vi "Autocross(2Lap).vi"() -> ()   [LabVIEW 2017]
uses:
  Control/AutocrossBestRecordIndicator.ctl
  Control/AutocrossCurrentRecordIndicator(2Lap).ctl
  Control/AutocrossState.ctl
  <vilib>/DAQmx/read.llb/DAQmx Read (Analog DBL 1Chan 1Samp).vi
  <vilib>/DAQmx/write.llb/DAQmx Write (Analog DBL 1Chan 1Samp).vi
  <vilib>/Utility/file.llb/Read Delimited Spreadsheet (string).vi
  <vilib>/DAQmx/create/channels.llb/DAQmx Create Channel (AO-Voltage-Basic).vi
  <vilib>/DAQmx/create/channels.llb/DAQmx Create Channel (AI-Voltage-Basic).vi
panel:
  out "Event Progress":string[][](table)
  in  "DeviceName":tag
  in  "OK Button":bool
  in  "Ready":bool
  in  "Retry":bool
  out "CurrentRecordIndicator":T1
  out "BestRecordIndicator":T2
  in  "Stop":bool
  # "2019 KSAE Formula Autocross Event"
  # "Lap1:"
  # "Lap2:"
  # "Total:"
  # "Entry:"
  # "#1"
  # "#2"
  # "#3"
  # "#4"
  # "Univ. :"
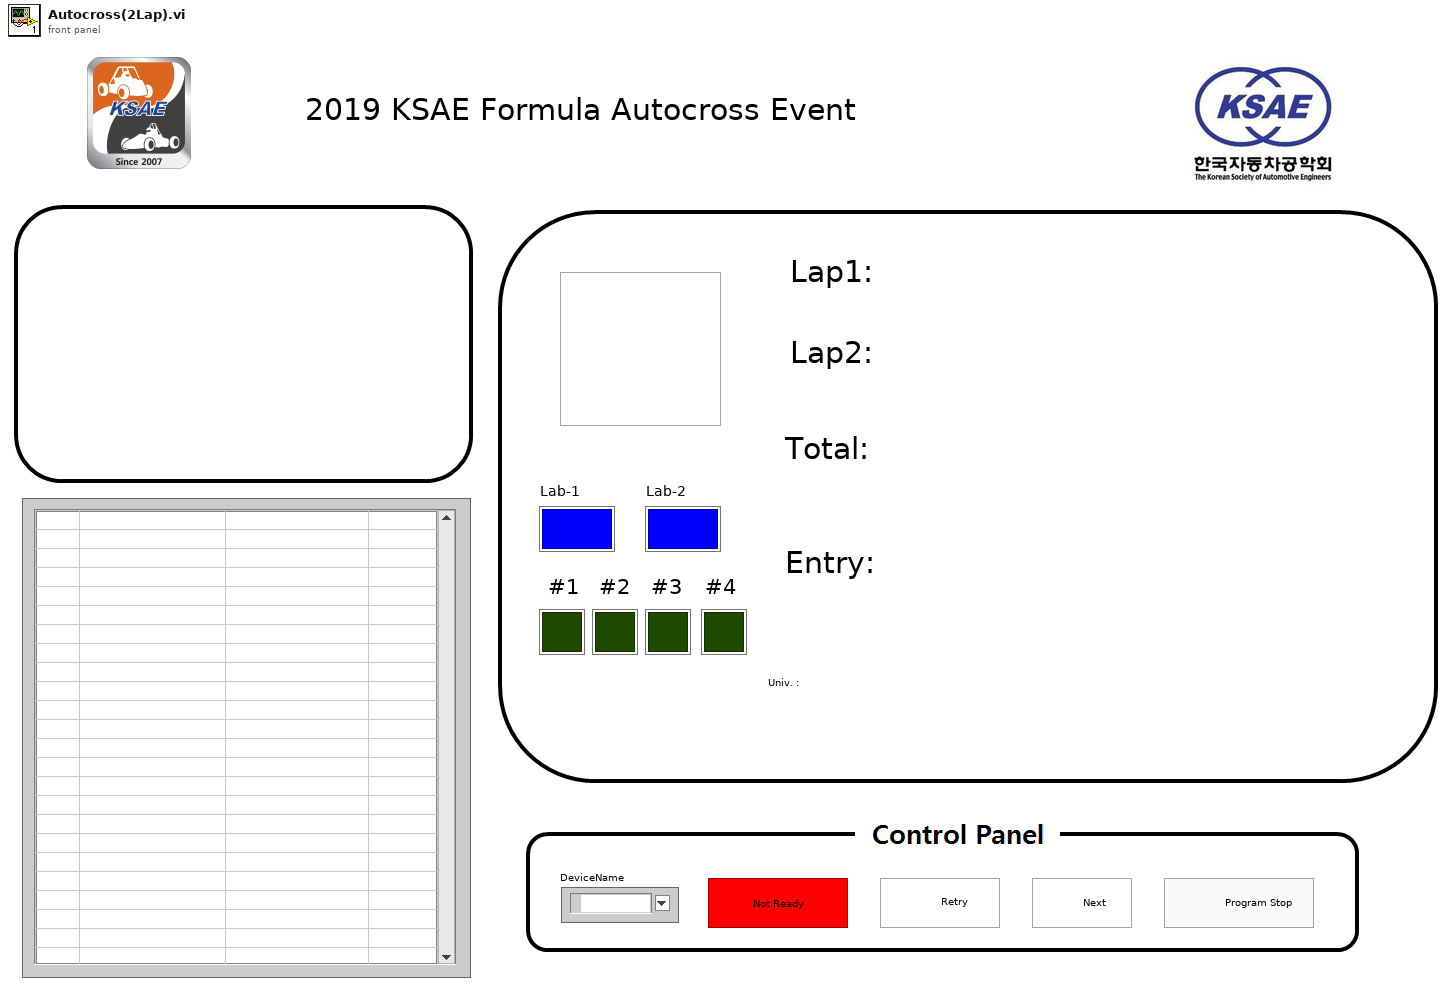
[diagram p1: front panel]
types:
  T1 = typedef "AutocrossCurrentRecordIndicator(2Lap).ctl" = cluster{"Lab1":string, "Lab2":string, "TotalLabTime":string, "CurrentEntry":string, "CurrentUniversity":string, "Flag":picture, "CurrentState":string, "LapProgress":cluster{"Lab-1":bool, "Lab-2":bool}, "EventCount":cluster{"Attempt-1":bool, "Attempt-2":bool, "Attempt-3":bool, "Attempt-4":bool}}
  T2 = typedef "AutocrossBestRecordIndicator.ctl" = cluster{"BestSchool":string, "BestEntry":string, "BestTime":string}
  T3 = typedef "AutocrossState.ctl" = enum16{"Initial", "InputInfomation", "Ready", "1lap", "2lap", "FinshRunning", "LogRecord", "RenewBestRecord", "ProgramStop"}
  T4 = cluster{"CurrentRecordIndicator":T1, "BestRecordIndicator":T2, "FlageData":cluster{"GreenFlag":picture, "BlueFlag":picture, "RedFlag":picture}, "1LapTime":i64, "2LapTime":i64, "TotalLabTime":i64, "InternalTime(1Lap)":i64, "InternalTime(2Lap)":i64, "State":T3, "EventProgressData":string[][], "EventCount":i32}
  T5 = cluster{"Attempt-1":bool, "Attempt-2":bool, "Attempt-3":bool, "Attempt-4":bool}
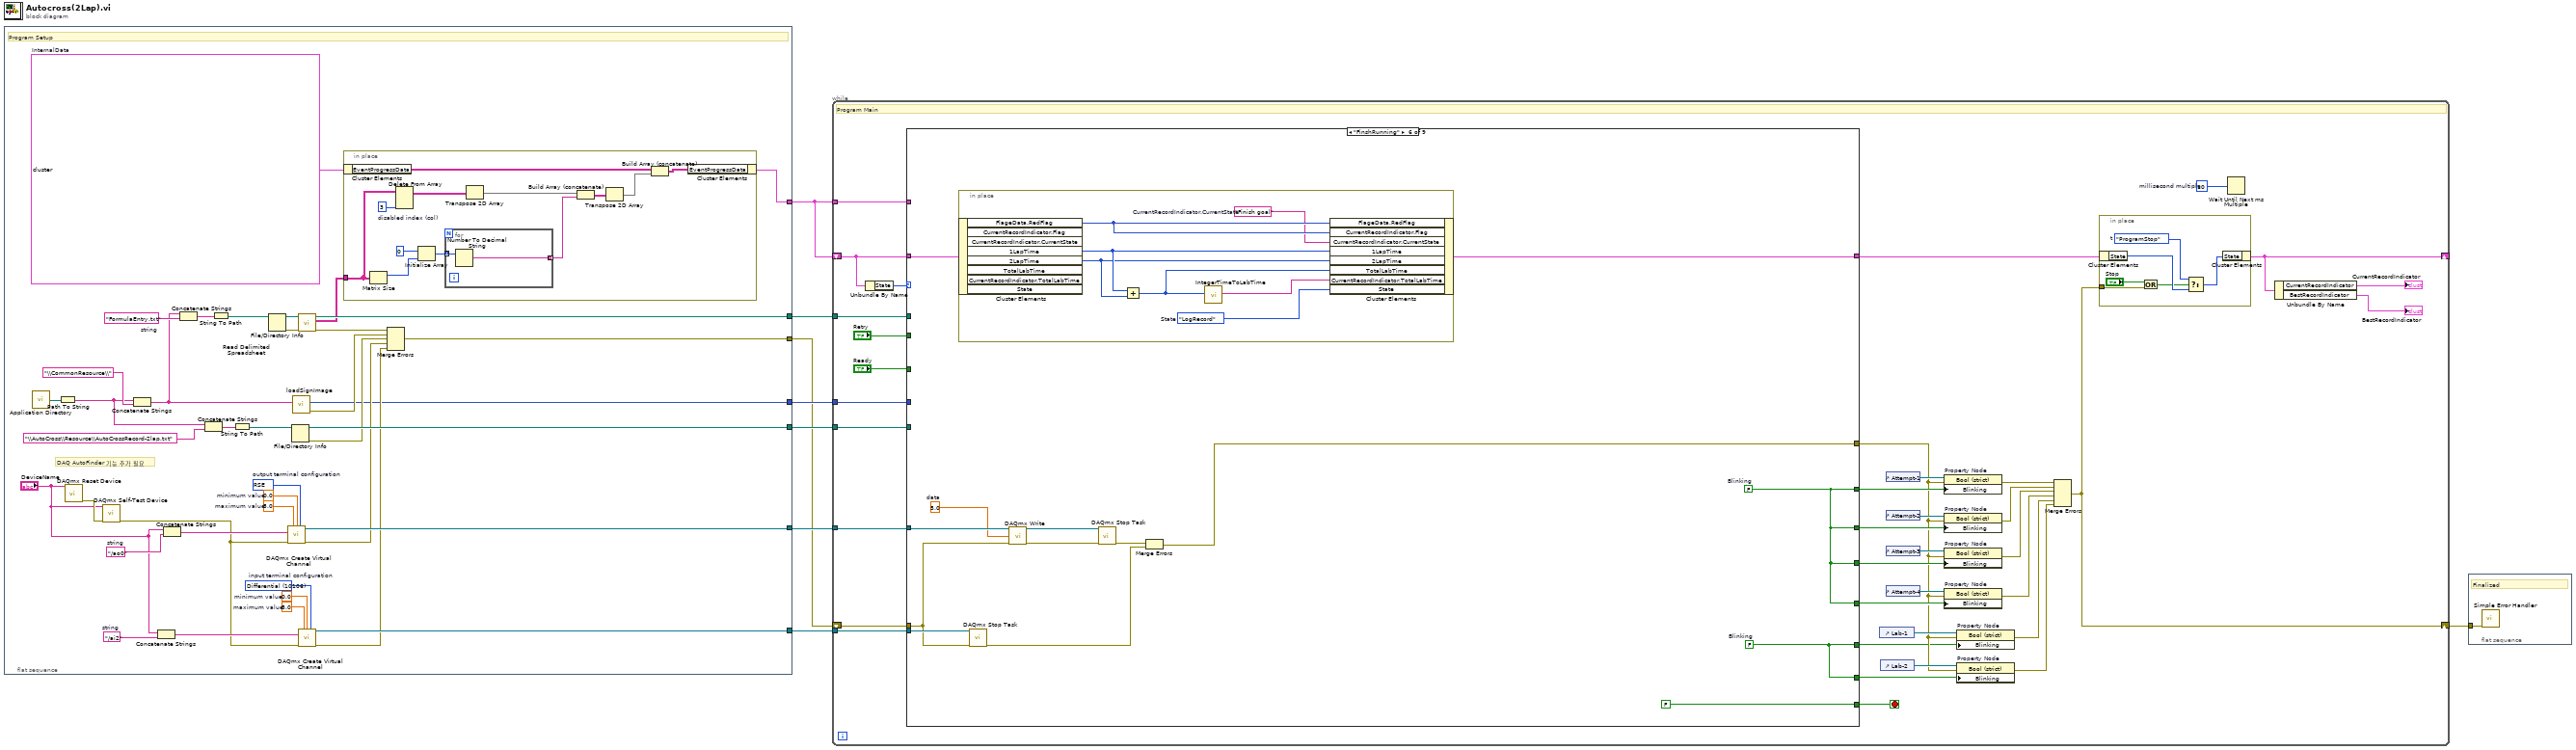
[diagram p0: block diagram]
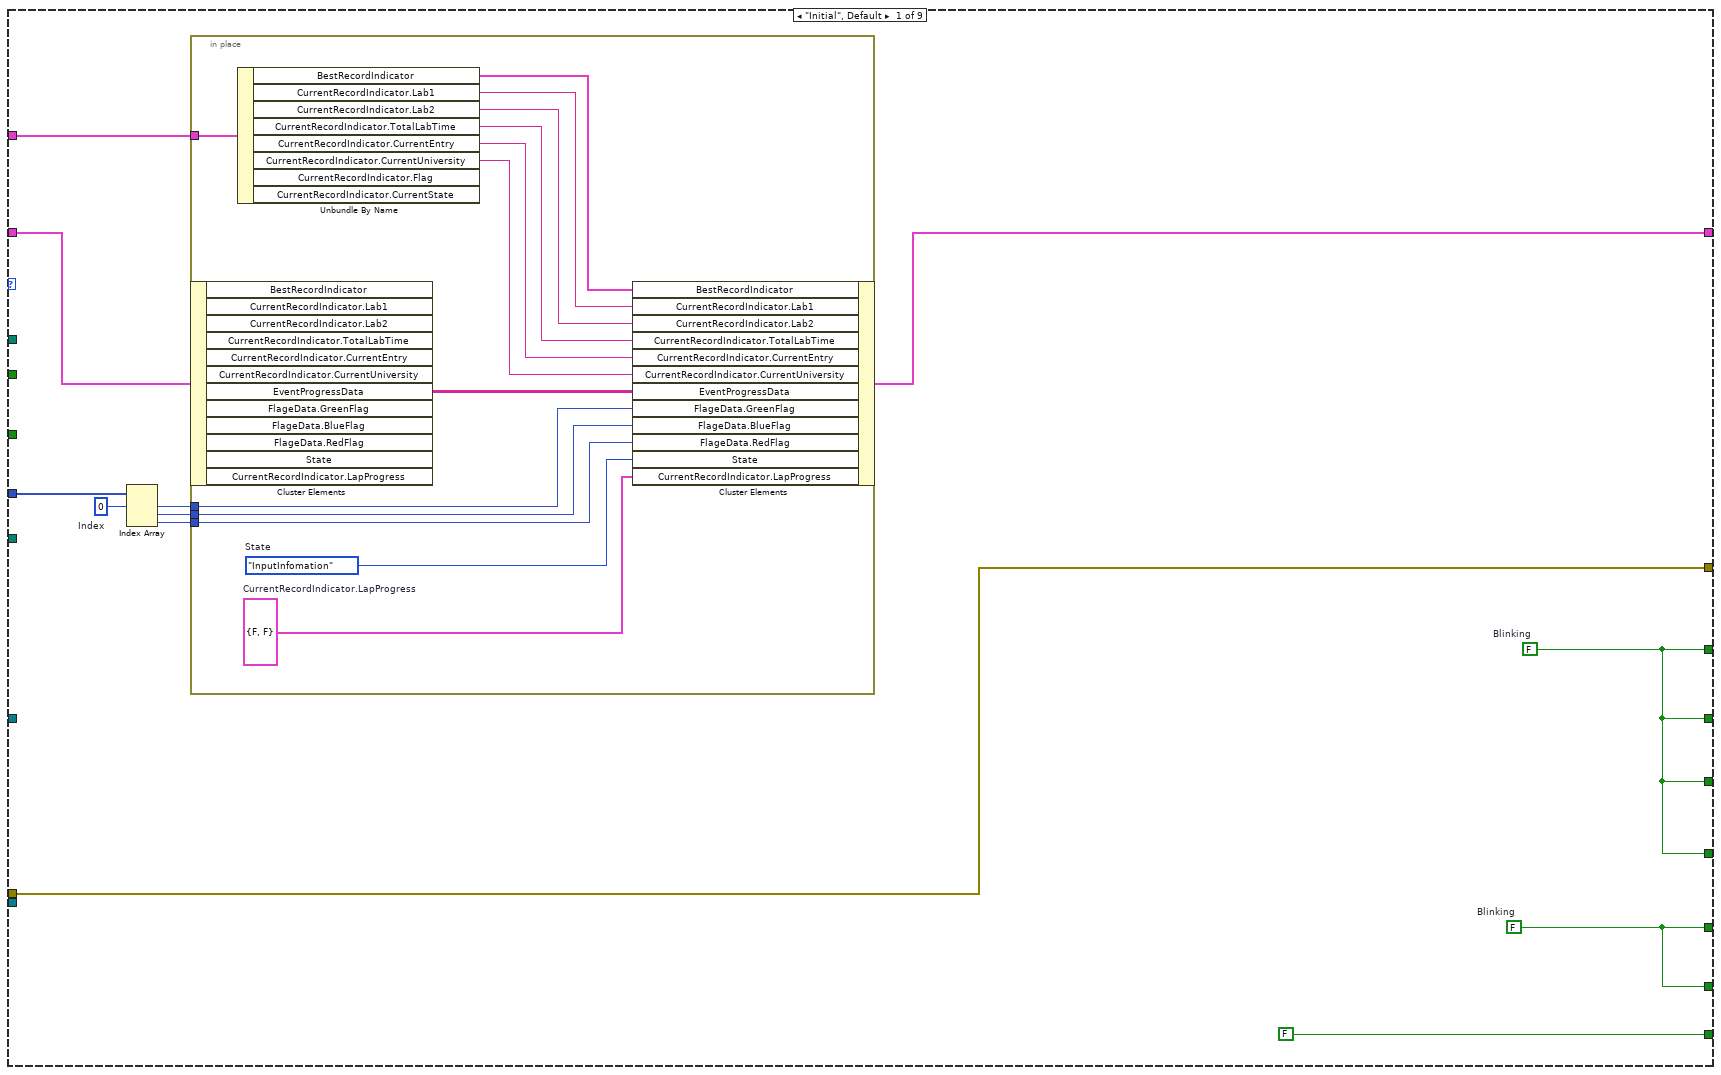
[diagram p2: hidden frame]
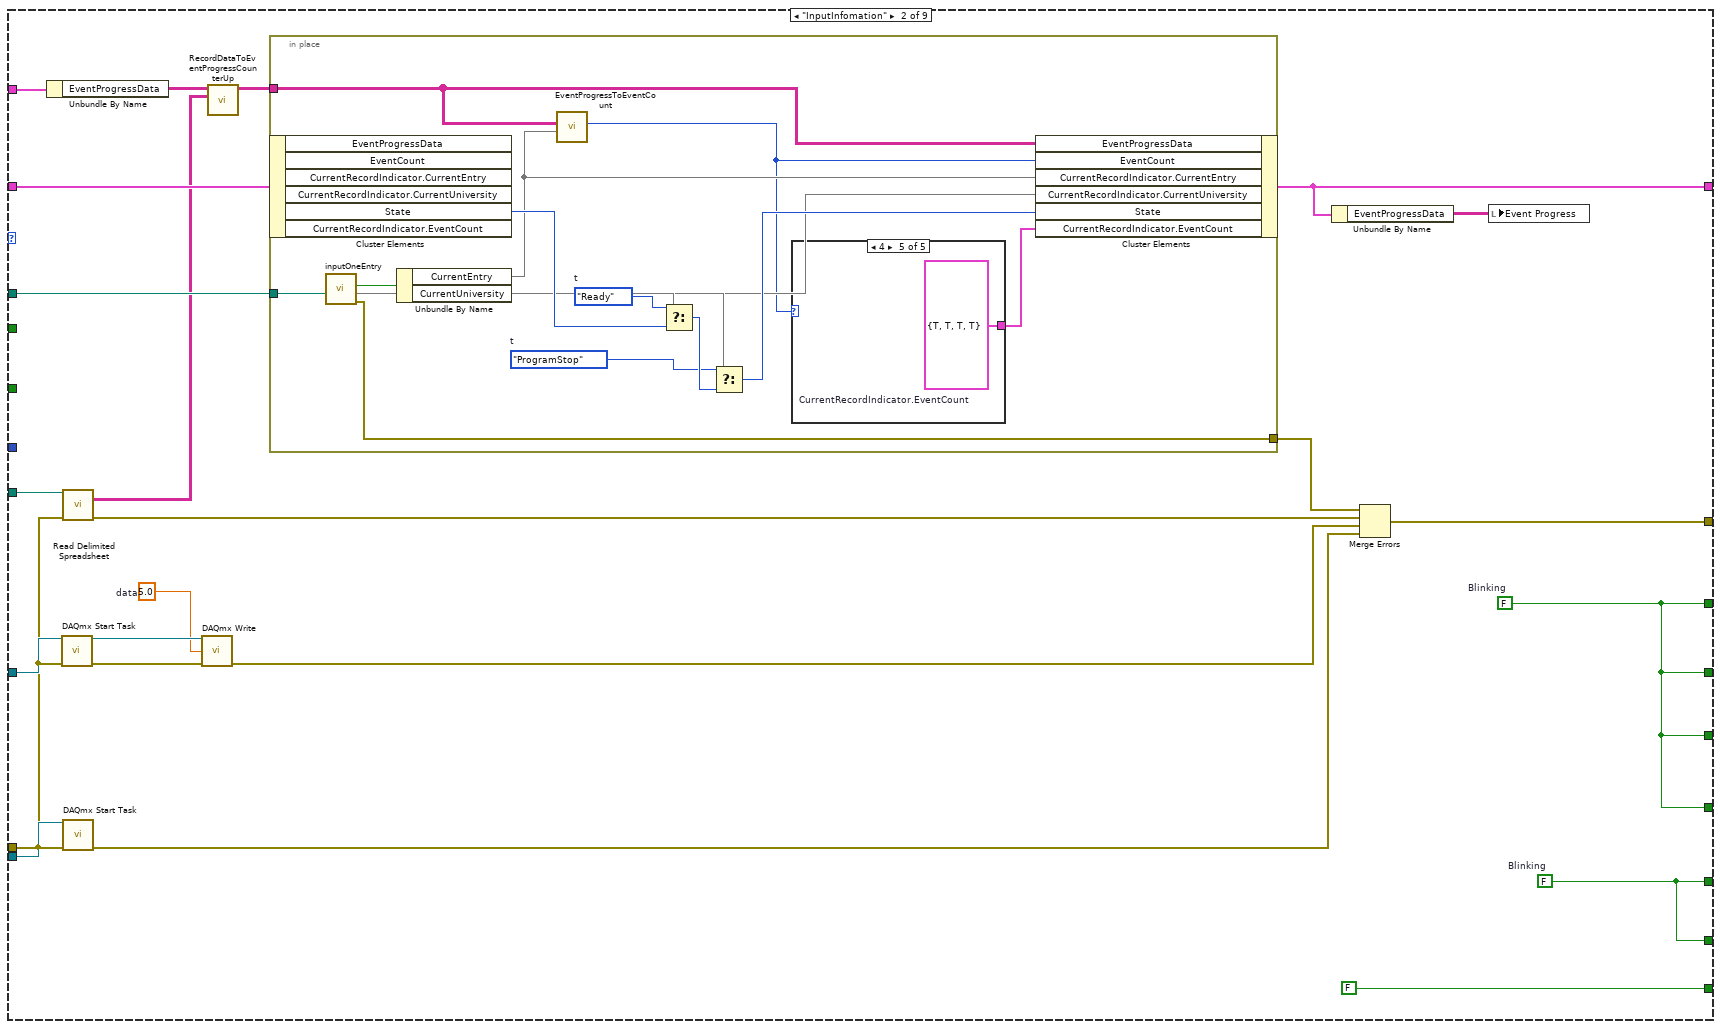
[diagram p3: hidden frame]
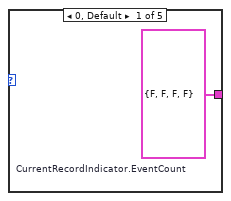
[diagram p4: hidden frame]
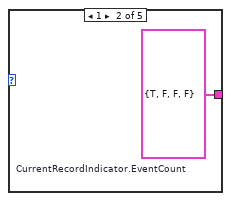
[diagram p5: hidden frame]
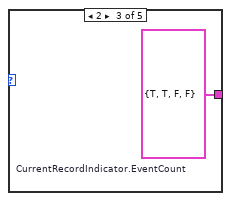
[diagram p6: hidden frame]
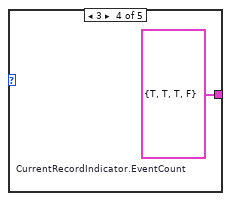
[diagram p7: hidden frame]
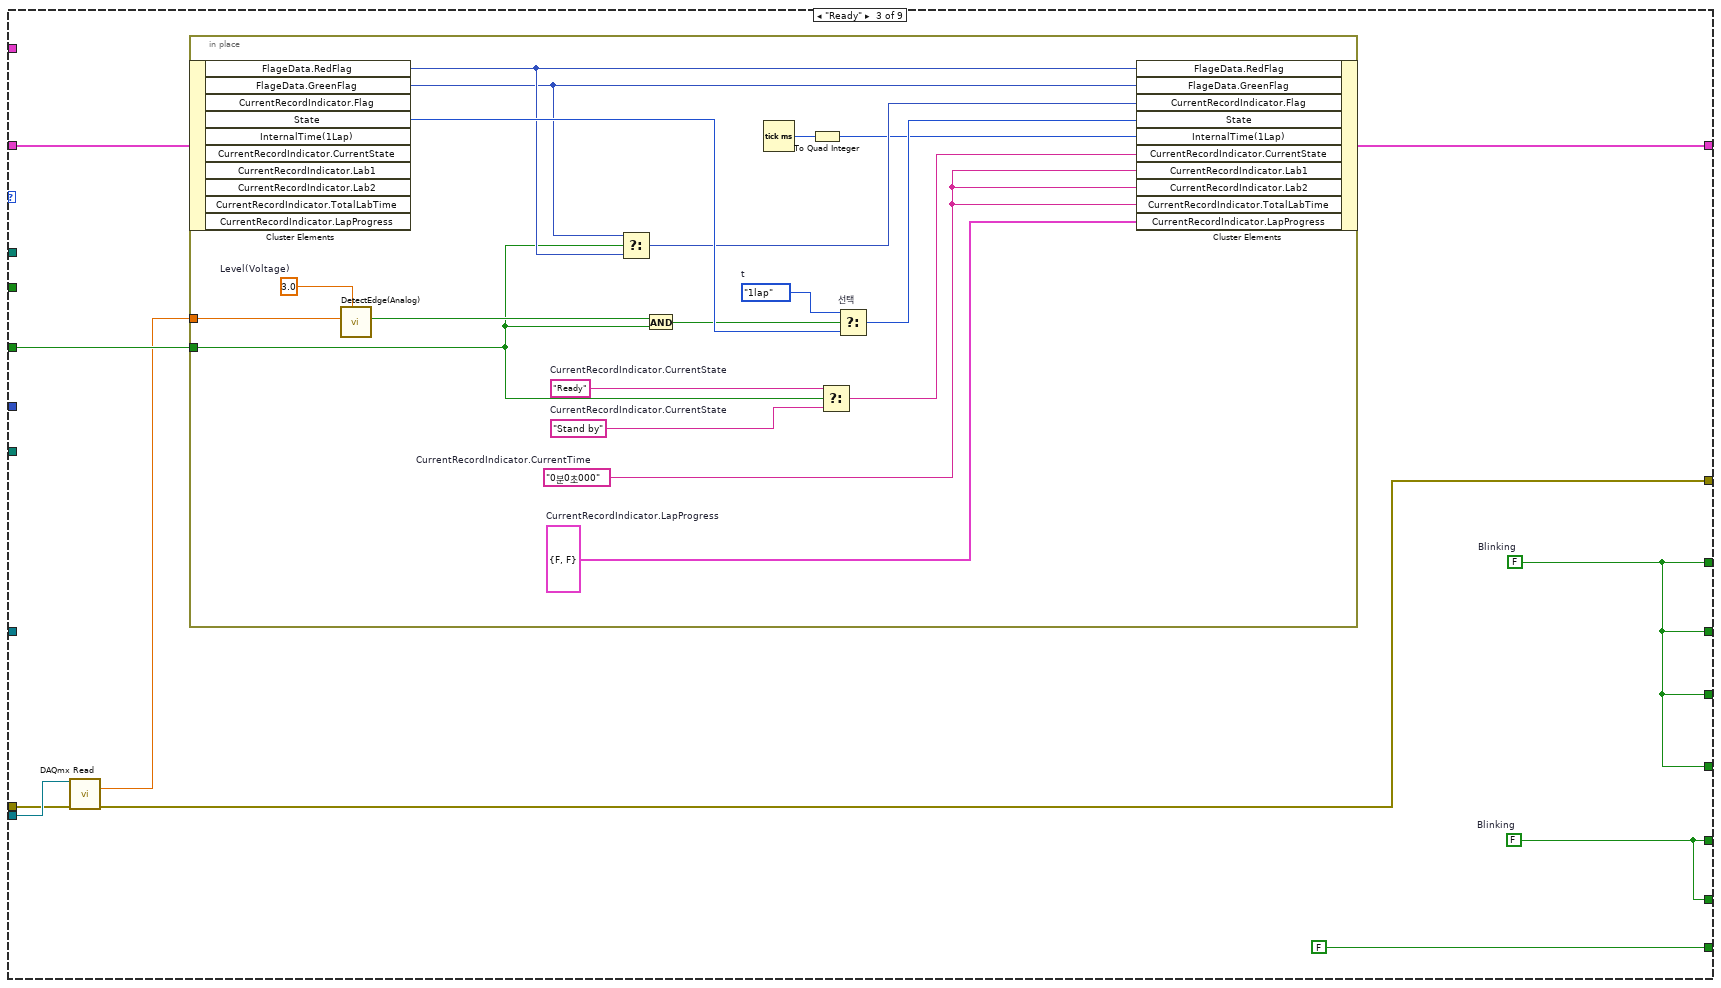
[diagram p8: hidden frame]
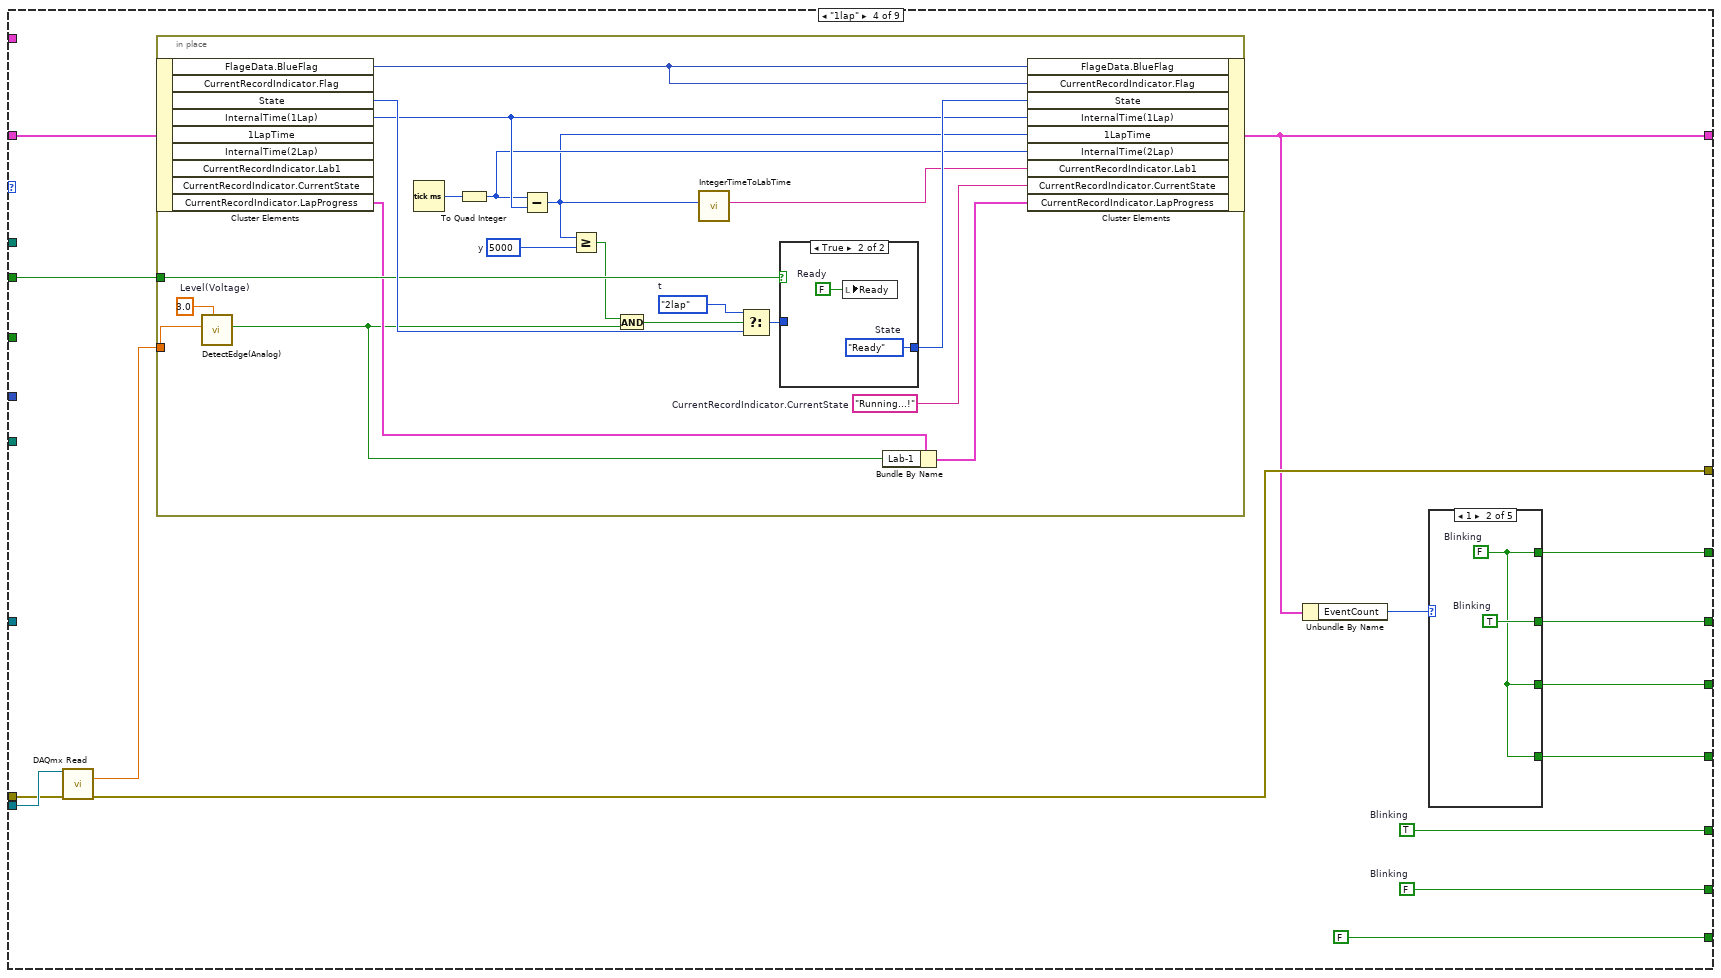
[diagram p9: hidden frame]
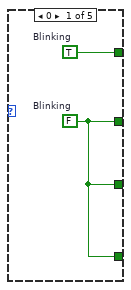
[diagram p10: hidden frame]
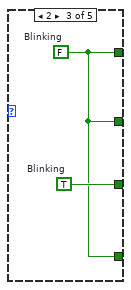
[diagram p11: hidden frame]
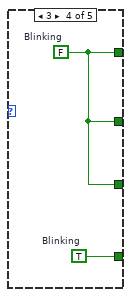
[diagram p12: hidden frame]
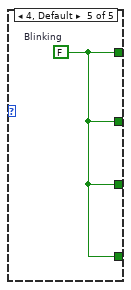
[diagram p13: hidden frame]
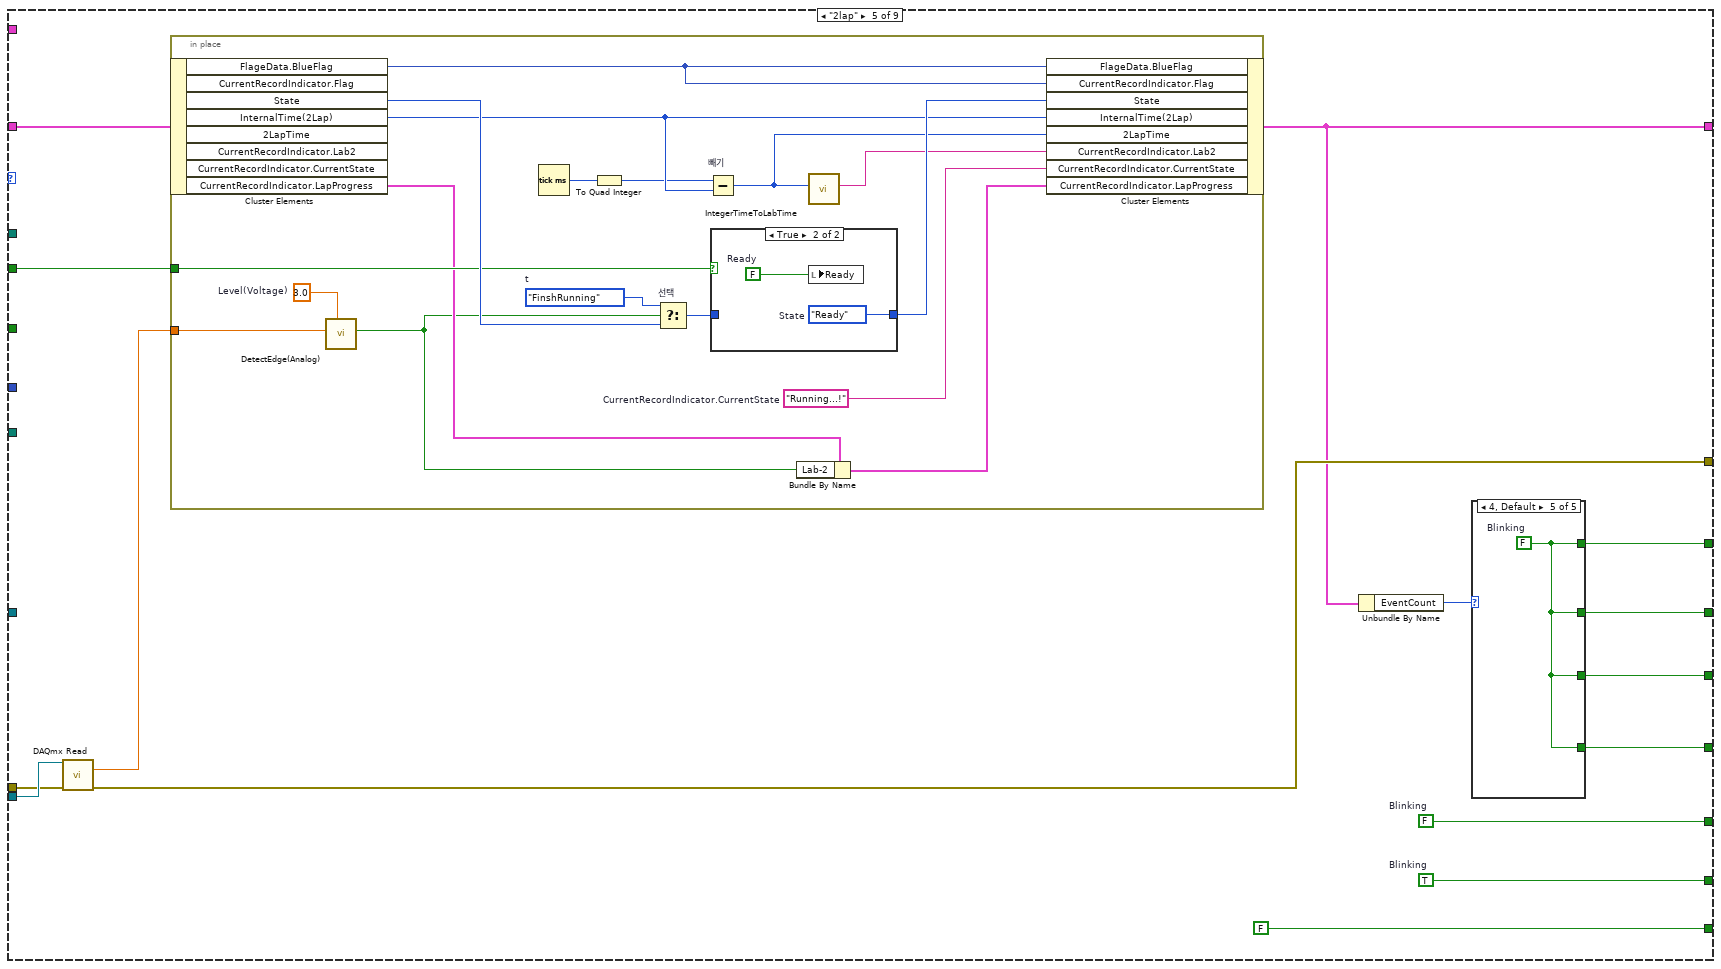
[diagram p15: hidden frame]
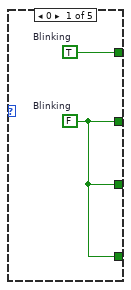
[diagram p16: hidden frame]
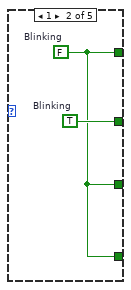
[diagram p17: hidden frame]
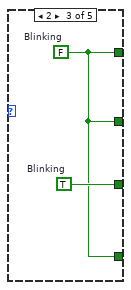
[diagram p18: hidden frame]
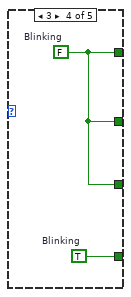
[diagram p19: hidden frame]
diagram:
  n1 = flat-sequence {
    tunnel: [w23] -> w7
    tunnel: [w46] -> w6
    tunnel: [w43] -> w5
    tunnel: [w25] -> w4
    tunnel: [w16] -> w3
    tunnel: [w9] -> w2
    tunnel: [w18] -> w1
    frame #0 {
      w24 = T4 {"CurrentRecordIndicator"={"Lab1"="", "Lab2"="", "TotalLabTime"="", "CurrentEntry"="", "CurrentUniversity"="", "Flag"=bytes[0], "CurrentState"="", "LapProgress"={"Lab-1"=FALSE, "Lab-2"=FALSE}, "EventCount"={"Attempt-1"=FALSE, "Attempt-2"=FALSE, "Attempt-3"=FALSE, "Attempt-4"=FALSE}}, "BestRecordIndicator"={"BestSchool"="", "BestEntry"="", "BestTime"=""}, "FlageData"={"GreenFlag"=bytes[0], "BlueFlag"=bytes[0], "RedFlag"=bytes[0]}, "1LapTime"=0, "2LapTime"=0, "TotalLabTime"=0, "InternalTime(1Lap)"=0, "InternalTime(2Lap)"=0, "State"=enum."Initial", "EventProgressData"=[["Entry ", "University", "Team", "Event Run "]], "EventCount"=0}  # InternalData
      w31 = "/ai2"  # string
      w32 = "/ao0"  # string
      w33 = "FormulaEntry.txt"  # string
      w40 = 10083 items=["Default"=-1, "RSE"=10083, "Differential"=10106, "Pseudodifferential"=12529]  # output terminal configuration
      w41 = 0.0  # minimum value
      w42 = 5.0  # maximum value
      w45 = 5.0  # maximum value
      w44 = 0.0  # minimum value
      w47 = 10106 items=["default"=-1, "RSE"=10083, "NRSE"=10078, "Differential"=10106, "Pseudodifferential"=12529]  # input terminal configuration
      # "DAQ AutoFinder 기능 추가 필요"
      # "Program Setup"
      n2 = call <vilib>:"Application Directory.vi"() -> ("Application Directory"=w39:path)
      n3 = Path To String(path=w39) -> (string=w35:string)
      n4 = call <vilib>:"DAQmx Reset Device.vi"("device in"="DeviceName") -> ("error out"=w12:errorcluster)  [unwired: 14 in]
      n5 = call <vilib>:"DAQmx Self-Test Device.vi"("device in"="DeviceName", "error in"=w12) -> ("error out"=w10:errorcluster)  [unwired: 13 in]
      n6 = Concatenate Strings "Concatenate Strings"(w35, "\\CommonResource\\") -> (w27:string)
      n7 = Concatenate Strings "Concatenate Strings"("DeviceName", w31) -> (w29:string)
      n8 = Concatenate Strings "Concatenate Strings"("DeviceName", w32) -> (w30:string)
      n9 = Concatenate Strings "Concatenate Strings"(w27, w33) -> (w34:string)
      n10 = Concatenate Strings "Concatenate Strings"(w35, "\\AutoCross\\Resource\\AutoCrossRecord-2lap.txt") -> (w37:string)
      n11 = String To Path(string=w34) -> (path=w26:path)
      n12 = String To Path(string=w37) -> (path=w28:path)
      n13 = File/Directory Info(path=w26) -> (path out=w17:path, error out=w15:errorcluster)  [unwired: 1 in, 5 out]
      n14 = call-poly <vilib>:"DAQmx Create Virtual Channel.vi"("maximum value"=w42, "minimum value"=w41, "output terminal configuration"=w40, "physical channels"=w30, "error in"=w10) -> ("task out"=w43:refnum<k21>, "error out"=w20:errorcluster)  [unwired: 9 in]
      n15 = File/Directory Info(path=w28) -> (path out=w25:path, error out=w21:errorcluster)  [unwired: 1 in, 5 out]
      n16 = call "loadSignImage.vi"("String"=w27) -> ("outputError"=w22:errorcluster, "SignImageOutput"=w9:picture[])  [unwired: 9 in]
      n17 = call-poly <vilib>:"Read Delimited Spreadsheet.vi"("file path (dialog if empty)"=w17, "error in (no error)"=w15) -> ("new file path (Not A Path if cancelled)"=w16:path, "all rows"=w13:string[][], "error out"=w14:errorcluster)  [unwired: 8 in, 3 out]
      n18 = call-poly <vilib>:"DAQmx Create Virtual Channel.vi"("maximum value"=w45, "minimum value"=w44, "input terminal configuration"=w47, "physical channels"=w29, "error in"=w10) -> ("task out"=w46:refnum<k21>, "error out"=w19:errorcluster)  [unwired: 9 in]
      n19 = in-place {
        in-place-border: w13 -> [w48]
        w56 = 3  # disabled index (col)
        n20 = in-place-cluster #1(w24) -> ("EventProgressData"=w50:string[][])
        n21 = Matrix Size(0:w48) -> (1:w59:i32)  [unwired: 1 out]
        n22 = Delete From Array "Delete From Array"(array=w48, index (col)=w56) -> (array with subset deleted=w55:string[][])  [unwired: 2 in, 1 out]
        n23 = Initialize Array "Initialize Array"(0, w59) -> (w57:i32[])
        n24 = for {
          tunnel: w57 -> [w61] mode=indexing
          tunnel: [w60] -> w53 mode=indexing
          n25 = Number To Decimal String(number=w61) -> (decimal integer string=w60:string)  [unwired: 1 in]
        }
        n26 = Transpose 2D Array(2D array=w55) -> (transposed array=w54:string[][])
        n27 = Build Array (concatenate) "Build Array"(w54, w53) -> (w52:string[][])
        n28 = Transpose 2D Array(2D array=w52) -> (transposed array=w51:string[][])
        n29 = Build Array (concatenate) "Build Array"(w50, w51) -> (w49:string[][])
        n30 = in-place-cluster #1("EventProgressData"=w49) -> (w23:T4)
      }
      n31 = Merge Errors "Merge Errors"(w14, w22, w21, w20, w19) -> (w18:errorcluster)
    }
  }
  n32 = while {
    tunnel: w6 -> [w98]
    shift-right: [w91] -> _
    shift-left: w7 -> [w95]
    shift-right: [w69] -> w8
    shift-left: w1 -> [w97]
    tunnel: w7 -> [w89]
    tunnel: w5 -> [w86]
    tunnel: w4 -> [w85]
    tunnel: w3 -> [w84]
    tunnel: w2 -> [w82]
    stop <- w90 stop-if-true
    w83 = u32 10  # millisecond multiple
    # "Program Main"
    n33 = Unbundle By Name(w95) -> ("State"=w96:T3)
    n34 = case shown="\"FinshRunning\"" w96 {
      tunnel: w98 -> [_ w151 w182 w215 w262 w305 _ _ w382]
      tunnel: w97 -> [w108 w133 w181 w214 w261 w294 w324 w362 w375]
      tunnel: w95 -> [w116 w152 w180 w213 w260 w304 w336 w364 w384]
      tunnel: [w115 w132 w179 w208 w251 w303 w315 w354 w383] -> w92
      tunnel: [FALSE FALSE FALSE FALSE FALSE FALSE FALSE FALSE TRUE] -> w90
      tunnel: [w108 w149 w178 w212 w259 w298 w321 w352 w378] -> w66
      tunnel: w89 -> [w109 w140 _ _ _ _ w320 _ _]
      tunnel: "Ready" -> [_ _ w177 _ _ _ _ _ _]
      tunnel: "Retry" -> [_ _ _ w211 w258 _ _ _ _]
      tunnel: w86 -> [_ w148 _ _ _ w301 _ _ w379]
      tunnel: w85 -> [_ w138 _ _ _ _ w327 w351 _]
      tunnel: w84 -> [_ w141 _ _ _ _ _ _ _]
      tunnel: w82 -> [w107 _ _ _ _ _ _ _ _]
      tunnel: [w106 w131 w174 w206 w255 w293 w314 w350 w376] -> w77
      tunnel: [w106 w131 w174 w205 w254 w293 w314 w350 w376] -> w76
      tunnel: [w106 w131 w174 w204 w253 w293 w314 w350 w376] -> w75
      tunnel: [w106 w131 w174 w203 w252 w293 w314 w350 w376] -> w74
      tunnel: [w105 w130 w173 w202 w249 w292 w313 w349 w374] -> w65
      tunnel: [w105 w130 w173 w201 w248 w292 w313 w349 w374] -> w64
      frame "Initial", Default {
        w105 = FALSE  # Blinking
        w106 = FALSE  # Blinking
        w110 = 0  # Index
        n35 = Index Array "Index Array"(array=w107, index #1=w110) -> (element #1=w113:picture, element #2=w112:picture, element #3=w111:picture)  [unwired: 2 in]
        n36 = in-place {
          in-place-border: w113 -> [w129]
          in-place-border: w112 -> [w128]
          in-place-border: w111 -> [w127]
          in-place-border: w109 -> [w125]
          w118 = cluster{"Lab1":bool, "Lab2":bool} {"Lab1"=FALSE, "Lab2"=FALSE}  # CurrentRecordIndicator.LapProgress
          w126 = AutocrossState."InputInfomation"  # State
          n37 = in-place-cluster #2(w116) -> ("EventProgressData"=w117:string[][])  [unwired: 11 out]
          n38 = Unbundle By Name(w125) -> ("BestRecordIndicator"=w124:T2, "CurrentRecordIndicator.Lab1"=w123:string, "CurrentRecordIndicator.Lab2"=w119:string, "CurrentRecordIndicator.TotalLabTime"=w122:string, "CurrentRecordIndicator.CurrentEntry"=w120:string, "CurrentRecordIndicator.CurrentUniversity"=w121:string)  [unwired: 2 out]
          n39 = in-place-cluster #2("BestRecordIndicator"=w124, "CurrentRecordIndicator.Lab1"=w123, "CurrentRecordIndicator.Lab2"=w119, "CurrentRecordIndicator.TotalLabTime"=w122, "CurrentRecordIndicator.CurrentEntry"=w120, "CurrentRecordIndicator.CurrentUniversity"=w121, "EventProgressData"=w117, "FlageData.GreenFlag"=w129, "FlageData.BlueFlag"=w128, "FlageData.RedFlag"=w127, "State"=w126, "CurrentRecordIndicator.LapProgress"=w118) -> (w115:T4)
        }
      }
      frame "InputInfomation" {
        w130 = FALSE  # Blinking
        w131 = FALSE  # Blinking
        w143 = 5.0  # data
        n40 = Unbundle By Name(w140) -> ("EventProgressData"=w139:string[][])
        n41 = call <vilib>:"DAQmx Start Task.vi"("task/channels in"=w148, "error in"=w133) -> ("task out"=w146:refnum<k21>, "error out"=w145:errorcluster)  [unwired: 12 in]
        n42 = call-poly <vilib>:"Read Delimited Spreadsheet.vi"("file path (dialog if empty)"=w138, "error in (no error)"=w133) -> ("all rows"=w137:string[][], "error out"=w135:errorcluster)  [unwired: 8 in, 4 out]
        n43 = call <vilib>:"DAQmx Start Task.vi"("task/channels in"=w151, "error in"=w133) -> ("error out"=w150:errorcluster)  [unwired: 12 in, 1 out]
        n44 = call-poly <vilib>:"DAQmx Write.vi"("task/channels in"=w146, "data"=w143, "error in"=w145) -> ("error out"=w144:errorcluster)  [unwired: 10 in, 2 out]
        n45 = call "RecordDataToEventProgressCounterUp.vi"("RecordData"=w137, "EventProgressDataInput"=w139) -> ("EventProgressDataOutput"=w136:string[][])  [unwired: 9 in]
        n46 = in-place {
          in-place-border: [w160] -> w147
          in-place-border: w141 -> [w157]
          in-place-border: w136 -> [w155]
          w164 = AutocrossState."ProgramStop"  # t
          w166 = AutocrossState."Ready"  # t
          n47 = in-place-cluster #3(w152) -> ("State"=w167:T3)  [unwired: 5 out]
          n48 = call "inputOneEntry.vi"(9:w157) -> ("outputError"=w160:errorcluster, "OKButtonOutput"=w159:bool, 4:w161, 6:w162)  [unwired: 5 in, 2 out]
          n49 = Unbundle By Name(w159) -> ("CurrentEntry"=w156, "CurrentUniversity"=w158)
          n50 = call "EventProgressToEventCount.vi"("CurrentEntry"=w156, "EventProgressDataInput"=w155) -> ("EventCount"=w154:i32)  [unwired: 9 in]
          n51 = Select(t=w166, s=w162, f=w167) -> (s? t:f=w165:T3)
          n52 = Select(t=w164, s=w161, f=w165) -> (s? t:f=w163:T3)
          n53 = case shown="4" w154 {
            tunnel: [w168 w169 w170 w171 w172] -> w153
            frame 0, Default {
              w168 = T5 {"Attempt-1"=FALSE, "Attempt-2"=FALSE, "Attempt-3"=FALSE, "Attempt-4"=FALSE}  # CurrentRecordIndicator.EventCount
            }
            frame 1 {
              w169 = T5 {"Attempt-1"=TRUE, "Attempt-2"=FALSE, "Attempt-3"=FALSE, "Attempt-4"=FALSE}  # CurrentRecordIndicator.EventCount
            }
            frame 2 {
              w170 = T5 {"Attempt-1"=TRUE, "Attempt-2"=TRUE, "Attempt-3"=FALSE, "Attempt-4"=FALSE}  # CurrentRecordIndicator.EventCount
            }
            frame 3 {
              w171 = T5 {"Attempt-1"=TRUE, "Attempt-2"=TRUE, "Attempt-3"=TRUE, "Attempt-4"=FALSE}  # CurrentRecordIndicator.EventCount
            }
            frame 4 {
              w172 = T5 {"Attempt-1"=TRUE, "Attempt-2"=TRUE, "Attempt-3"=TRUE, "Attempt-4"=TRUE}  # CurrentRecordIndicator.EventCount
            }
          }
          n54 = in-place-cluster #3("EventProgressData"=w155, "EventCount"=w154, "CurrentRecordIndicator.CurrentEntry"=w156, "CurrentRecordIndicator.CurrentUniversity"=w158, "State"=w163, "CurrentRecordIndicator.EventCount"=w153) -> (w132:T4)
        }
        n55 = Unbundle By Name(w132) -> ("EventProgressData"=w134:string[][])
        n56 = Merge Errors "Merge Errors"(w147, w135, w144, w150) -> (w149:errorcluster)
        n57 = local write "Event Progress"(w134) -> ()
      }
      frame "Ready" {
        w173 = FALSE  # Blinking
        w174 = FALSE  # Blinking
        n58 = call-poly <vilib>:"DAQmx Read.vi"("task/channels in"=w182, "error in"=w181) -> ("data"=w176:dbl, "error out"=w178:errorcluster)  [unwired: 11 in, 1 out]
        n59 = in-place {
          in-place-border: w176 -> [w196]
          in-place-border: w177 -> [w190]
          w186 = cluster{"Lab1":bool, "Lab2":bool} {"Lab1"=FALSE, "Lab2"=FALSE}  # CurrentRecordIndicator.LapProgress
          w187 = "Stand by"  # CurrentRecordIndicator.CurrentState
          w191 = 3.0  # Level(Voltage)
          w184 = "0분0초000"  # CurrentRecordIndicator.CurrentTime
          w188 = "Ready"  # CurrentRecordIndicator.CurrentState
          w198 = AutocrossState."1lap"  # t
          n60 = in-place-cluster #4(w180) -> ("FlageData.RedFlag"=w193:picture, "FlageData.GreenFlag"=w192:picture, "State"=w200:T3)  [unwired: 7 out]
          n61 = call "DetectEdge(Analog).vi"("Level(Voltage)"=w191, "Voltage"=w196) -> ("DetectedEdge"=w197:bool)  [unwired: 9 in]
          n62 = Select(t=w192, s=w190, f=w193) -> (s? t:f=w194:picture)
          n63 = And(x=w197, y=w190) -> (x .and. y?=w195:bool)
          n64 = Tick Count (ms)() -> (millisecond timer value=w185:u32)
          n65 = To Quad Integer(1:w185) -> (0:w183:i64)
          n66 = Select(t=w188, s=w190, f=w187) -> (s? t:f=w189:string)
          n67 = Select "선택"(t=w198, s=w195, f=w200) -> (s? t:f=w199:T3)
          n68 = in-place-cluster #4("FlageData.RedFlag"=w193, "FlageData.GreenFlag"=w192, "CurrentRecordIndicator.Flag"=w194, "State"=w199, "InternalTime(1Lap)"=w183, "CurrentRecordIndicator.CurrentState"=w189, "CurrentRecordIndicator.Lab1"=w184, "CurrentRecordIndicator.Lab2"=w184, "CurrentRecordIndicator.TotalLabTime"=w184, "CurrentRecordIndicator.LapProgress"=w186) -> (w179:T4)
        }
      }
      frame "1lap" {
        w201 = FALSE  # Blinking
        w202 = TRUE  # Blinking
        n69 = call-poly <vilib>:"DAQmx Read.vi"("task/channels in"=w215, "error in"=w214) -> ("data"=w210:dbl, "error out"=w212:errorcluster)  [unwired: 11 in, 1 out]
        n70 = in-place {
          in-place-border: w211 -> [w240]
          in-place-border: w210 -> [w237]
          w227 = i64 5000  # y
          w236 = 3.0  # Level(Voltage)
          w241 = "Running...!"  # CurrentRecordIndicator.CurrentState
          w243 = AutocrossState."2lap"  # t
          n71 = in-place-cluster #5(w213) -> ("FlageData.BlueFlag"=w242:picture, "State"=w244:T3, "InternalTime(1Lap)"=w231:i64, "CurrentRecordIndicator.LapProgress"=w235:cluster{"Lab-1":bool, "Lab-2":bool})  [unwired: 5 out]
          n72 = call "DetectEdge(Analog).vi"("Level(Voltage)"=w236, "Voltage"=w237) -> ("DetectedEdge"=w233:bool)  [unwired: 9 in]
          n73 = Tick Count (ms)() -> (millisecond timer value=w232:u32)
          n74 = To Quad Integer(1:w232) -> (0:w229:i64)
          n75 = Subtract(x=w229, y=w231) -> (x-y=w228:i64)
          n76 = Greater Or Equal?(x=w228, y=w227) -> (x >= y?=w225:bool)
          n77 = And(x=w225, y=w233) -> (x .and. y?=w226:bool)
          n78 = call "IntegerTimeToLabTime.vi"("inputTime(msec)"=w228) -> ("outputTime(mm-ss-sss)"=w230:string)  [unwired: 10 in]
          n79 = Select(t=w243, s=w226, f=w244) -> (s? t:f=w239:T3)
          n80 = case shown="True" w240 {
            tunnel: w239 -> [w245 _]
            tunnel: [w245 w246] -> w238
            frame False {
            }
            frame True {
              w246 = AutocrossState."Ready"  # State
              w247 = FALSE  # Ready
              n81 = local write "Ready"(w247) -> ()
            }
          }
          n82 = Bundle By Name(cluster=w235, "Lab-1"=w233) -> (w234:cluster{"Lab-1":bool, "Lab-2":bool})
          n83 = in-place-cluster #5("FlageData.BlueFlag"=w242, "CurrentRecordIndicator.Flag"=w242, "State"=w238, "InternalTime(1Lap)"=w231, "1LapTime"=w228, "InternalTime(2Lap)"=w229, "CurrentRecordIndicator.Lab1"=w230, "CurrentRecordIndicator.CurrentState"=w241, "CurrentRecordIndicator.LapProgress"=w234) -> (w208:T4)
        }
        n84 = Unbundle By Name(w208) -> ("EventCount"=w207:i32)
        n85 = case shown="1" w207 {
          tunnel: [w217 w218 w220 w222 w224] -> w206
          tunnel: [w216 w219 w220 w222 w224] -> w205
          tunnel: [w216 w218 w221 w222 w224] -> w204
          tunnel: [w216 w218 w220 w223 w224] -> w203
          frame 0 {
            w216 = FALSE  # Blinking
            w217 = TRUE  # Blinking
          }
          frame 1 {
            w219 = TRUE  # Blinking
            w218 = FALSE  # Blinking
          }
          frame 2 {
            w221 = TRUE  # Blinking
            w220 = FALSE  # Blinking
          }
          frame 3 {
            w223 = TRUE  # Blinking
            w222 = FALSE  # Blinking
          }
          frame 4, Default {
            w224 = FALSE  # Blinking
          }
        }
      }
      frame "2lap" {
        w248 = TRUE  # Blinking
        w249 = FALSE  # Blinking
        n86 = call-poly <vilib>:"DAQmx Read.vi"("task/channels in"=w262, "error in"=w261) -> ("data"=w257:dbl, "error out"=w259:errorcluster)  [unwired: 11 in, 1 out]
        n87 = in-place {
          in-place-border: w258 -> [w284]
          in-place-border: w257 -> [w281]
          w280 = 3.0  # Level(Voltage)
          w285 = "Running...!"  # CurrentRecordIndicator.CurrentState
          w287 = AutocrossState."FinshRunning"  # t
          n88 = in-place-cluster #6(w260) -> ("FlageData.BlueFlag"=w286:picture, "State"=w288:T3, "InternalTime(2Lap)"=w275:i64, "CurrentRecordIndicator.LapProgress"=w279:cluster{"Lab-1":bool, "Lab-2":bool})  [unwired: 4 out]
          n89 = call "DetectEdge(Analog).vi"("Level(Voltage)"=w280, "Voltage"=w281) -> ("DetectedEdge"=w277:bool)  [unwired: 9 in]
          n90 = Tick Count (ms)() -> (millisecond timer value=w276:u32)
          n91 = To Quad Integer(1:w276) -> (0:w272:i64)
          n92 = Select "선택"(t=w287, s=w277, f=w288) -> (s? t:f=w283:T3)
          n93 = Subtract "빼기"(x=w272, y=w275) -> (x-y=w273:i64)
          n94 = case shown="True" w284 {
            tunnel: w283 -> [w289 _]
            tunnel: [w289 w290] -> w282
            frame False {
            }
            frame True {
              w290 = AutocrossState."Ready"  # State
              w291 = FALSE  # Ready
              n95 = local write "Ready"(w291) -> ()
            }
          }
          n96 = Bundle By Name(cluster=w279, "Lab-2"=w277) -> (w278:cluster{"Lab-1":bool, "Lab-2":bool})
          n97 = call "IntegerTimeToLabTime.vi"("inputTime(msec)"=w273) -> ("outputTime(mm-ss-sss)"=w274:string)  [unwired: 10 in]
          n98 = in-place-cluster #6("FlageData.BlueFlag"=w286, "CurrentRecordIndicator.Flag"=w286, "State"=w282, "InternalTime(2Lap)"=w275, "2LapTime"=w273, "CurrentRecordIndicator.Lab2"=w274, "CurrentRecordIndicator.CurrentState"=w285, "CurrentRecordIndicator.LapProgress"=w278) -> (w251:T4)
        }
        n99 = Unbundle By Name(w251) -> ("EventCount"=w250:i32)
        n100 = case shown="4, Default" w250 {
          tunnel: [w264 w265 w267 w269 w271] -> w255
          tunnel: [w263 w266 w267 w269 w271] -> w254
          tunnel: [w263 w265 w268 w269 w271] -> w253
          tunnel: [w263 w265 w267 w270 w271] -> w252
          frame 0 {
            w263 = FALSE  # Blinking
            w264 = TRUE  # Blinking
          }
          frame 1 {
            w266 = TRUE  # Blinking
            w265 = FALSE  # Blinking
          }
          frame 2 {
            w268 = TRUE  # Blinking
            w267 = FALSE  # Blinking
          }
          frame 3 {
            w270 = TRUE  # Blinking
            w269 = FALSE  # Blinking
          }
          frame 4, Default {
            w271 = FALSE  # Blinking
          }
        }
      }
      frame "FinshRunning" {
        w292 = FALSE  # Blinking
        w293 = FALSE  # Blinking
        w296 = 5.0  # data
        n101 = in-place {
          w310 = AutocrossState."LogRecord"  # State
          w311 = "Finish goal"  # CurrentRecordIndicator.CurrentState
          n102 = in-place-cluster #7(w304) -> ("FlageData.RedFlag"=w312:picture, "1LapTime"=w308:i64, "2LapTime"=w307:i64)  [unwired: 5 out]
          n103 = Add(x=w308, y=w307) -> (x+y=w306:i64)
          n104 = call "IntegerTimeToLabTime.vi"("inputTime(msec)"=w306) -> ("outputTime(mm-ss-sss)"=w309:string)  [unwired: 10 in]
          n105 = in-place-cluster #7("FlageData.RedFlag"=w312, "CurrentRecordIndicator.Flag"=w312, "CurrentRecordIndicator.CurrentState"=w311, "1LapTime"=w308, "2LapTime"=w307, "TotalLabTime"=w306, "CurrentRecordIndicator.TotalLabTime"=w309, "State"=w310) -> (w303:T4)
        }
        n106 = call <vilib>:"DAQmx Stop Task.vi"("task/channels in"=w305, "error in"=w294) -> ("error out"=w302:errorcluster)  [unwired: 12 in, 1 out]
        n107 = call-poly <vilib>:"DAQmx Write.vi"("task/channels in"=w301, "data"=w296, "error in"=w294) -> ("task out"=w300:refnum<k21>, "error out"=w299:errorcluster)  [unwired: 10 in, 1 out]
        n108 = call <vilib>:"DAQmx Stop Task.vi"("task/channels in"=w300, "error in"=w299) -> ("error out"=w297:errorcluster)  [unwired: 12 in, 1 out]
        n109 = Merge Errors "Merge Errors"(w297, w302) -> (w298:errorcluster)
      }
      frame "LogRecord" {
        w313 = FALSE  # Blinking
        w314 = FALSE  # Blinking
        w328 = "\t"  # Tab Constant
        # "Logged File Format\nCurrentEntry <tab> CurrentUniversity <tab> CurrentLab1 <tab> CurrentLab2 <tab> CurrentTotalLabTime <tab> Internal Time"
        n110 = in-place {
          in-place-border: [w347] -> w332
          w348 = AutocrossState."RenewBestRecord"  # State
          n111 = in-place-cluster #8(w336) -> ("TotalLabTime"=w347:i64)  [unwired: 1 out]
          n112 = in-place-cluster #8("TotalLabTime"=w347, "State"=w348) -> (w318:T4)
        }
        n113 = Unbundle By Name(w336) -> ("CurrentRecordIndicator.CurrentEntry"=w326:string, "CurrentRecordIndicator.CurrentUniversity"=w335:string, "CurrentRecordIndicator.Lab1"=w334:string, "CurrentRecordIndicator.Lab2"=w329:string, "CurrentRecordIndicator.TotalLabTime"=w331:string)
        n114 = Unbundle By Name(w320) -> ("EventProgressData"=w319:string[][])
        n115 = Number To Decimal String(number=w332) -> (decimal integer string=w330:string)  [unwired: 1 in]
        n116 = Concatenate Strings "Concatenate Strings"(w326, w328, w335, w328, w334, w328, w329, w328, w331, w328, w330) -> (w333:string)
        n117 = call "AddRecordFile.vi"("에러 입력"=w324, "LabTime"=w333, "파일 경로(대화 상자 사용)"=w327) -> ("에러 출력"=w322:errorcluster, "경로"=w323:path)  [unwired: 7 in]
        n118 = call-poly <vilib>:"Read Delimited Spreadsheet.vi"("file path (dialog if empty)"=w323, "error in (no error)"=w322) -> ("all rows"=w317:string[][], "error out"=w321:errorcluster)  [unwired: 8 in, 4 out]
        n119 = call "RecordDataToEventProgressCounterUp.vi"("RecordData"=w317, "EventProgressDataInput"=w319) -> ("EventProgressDataOutput"=w316:string[][])  [unwired: 9 in]
        n120 = in-place {
          in-place-border: w316 -> [w341]
          n121 = in-place-cluster #9(w318) -> ("CurrentRecordIndicator.CurrentEntry"=w340:string)  [unwired: 3 out]
          n122 = call "EventProgressToEventCount.vi"("CurrentEntry"=w340, "EventProgressDataInput"=w341) -> ("EventCount"=w339:i32)  [unwired: 9 in]
          n123 = case shown="4" w339 {
            tunnel: [w342 w343 w344 w345 w346] -> w338
            frame 0, Default {
              w342 = T5 {"Attempt-1"=FALSE, "Attempt-2"=FALSE, "Attempt-3"=FALSE, "Attempt-4"=FALSE}  # CurrentRecordIndicator.EventCount
            }
            frame 1 {
              w343 = T5 {"Attempt-1"=TRUE, "Attempt-2"=FALSE, "Attempt-3"=FALSE, "Attempt-4"=FALSE}  # CurrentRecordIndicator.EventCount
            }
            frame 2 {
              w344 = T5 {"Attempt-1"=TRUE, "Attempt-2"=TRUE, "Attempt-3"=FALSE, "Attempt-4"=FALSE}  # CurrentRecordIndicator.EventCount
            }
            frame 3 {
              w345 = T5 {"Attempt-1"=TRUE, "Attempt-2"=TRUE, "Attempt-3"=TRUE, "Attempt-4"=FALSE}  # CurrentRecordIndicator.EventCount
            }
            frame 4 {
              w346 = T5 {"Attempt-1"=TRUE, "Attempt-2"=TRUE, "Attempt-3"=TRUE, "Attempt-4"=TRUE}  # CurrentRecordIndicator.EventCount
            }
          }
          n124 = in-place-cluster #9("EventProgressData"=w341, "CurrentRecordIndicator.CurrentEntry"=w340, "EventCount"=w339, "CurrentRecordIndicator.EventCount"=w338) -> (w315:T4)
        }
        n125 = Unbundle By Name(w315) -> ("EventProgressData"=→"Event Progress":string[][])
      }
      frame "RenewBestRecord" {
        w349 = FALSE  # Blinking
        w350 = FALSE  # Blinking
        w356 = 5  # IndexColumn
        w357 = 0  # Index
        n126 = call "ReadBestRecord.vi"("IndexColumn"=w356, "ErrorInput"=w362, "FilepathInput"=w351) -> ("ErrorOutput"=w353:errorcluster, "Data"=w361:string[])  [unwired: 6 in, 1 out]
        n127 = flat-sequence {
          tunnel: w353 -> [w365]
          tunnel: [w365] -> w352
          frame #0 {
            w366 = FALSE  # Ready
            n128 = local write "Ready"(w366) -> ()
          }
        }
        n129 = Index Array "Index Array"(array=w361, index #1=w357) -> (element #1=w360:string, element #2=w359:string, element #3=w358:string)  [unwired: 2 in]
        n130 = in-place {
          in-place-border: w360 -> [w373]
          in-place-border: w359 -> [w372]
          in-place-border: w358 -> [w371]
          n131 = in-place-cluster #10(w364) -> ()  [unwired: 3 out]
          n132 = in-place-cluster #10("BestRecordIndicator.BestEntry"=w373, "BestRecordIndicator.BestSchool"=w372, "BestRecordIndicator.BestTime"=w371) -> (w355:T4)
        }
        n133 = in-place {
          w369 = AutocrossState."InputInfomation"  # State
          n134 = in-place-cluster #11(w355) -> ("State"=w367:T3)
          n135 = Select(t=w369, s="OK Button", f=w367) -> (s? t:f=w368:T3)
          n136 = in-place-cluster #11("State"=w368) -> (w354:T4)
        }
      }
      frame "ProgramStop" {
        w374 = FALSE  # Blinking
        w376 = FALSE  # Blinking
        n137 = call <vilib>:"DAQmx Clear Task.vi"("task in"=w379, "error in"=w375) -> ("error out"=w377:errorcluster)  [unwired: 13 in]
        n138 = call <vilib>:"DAQmx Clear Task.vi"("task in"=w382, "error in"=w375) -> ("error out"=w381:errorcluster)  [unwired: 13 in]
        n139 = in-place {
          w389 = "Halted Program"  # CurrentRecordIndicator.CurrentState
          n140 = in-place-cluster #12(w384) -> ("FlageData.RedFlag"=w388:picture)  [unwired: 2 out]
          n141 = in-place-cluster #12("FlageData.RedFlag"=w388, "CurrentRecordIndicator.Flag"=w388, "CurrentRecordIndicator.CurrentState"=w389) -> (w383:T4)
        }
        n142 = flat-sequence {
          tunnel: w381 -> [w387]
          tunnel: [w387] -> w380
          frame #0 {
            w386 = FALSE  # Ready
            n143 = local write "Ready"(w386) -> ()
          }
        }
        n144 = Merge Errors "Merge Errors"(w377, w380) -> (w378:errorcluster)
      }
    }
    n145 = control-ref of="Lab-1"() -> (w68:refnum<vi>)
    n146 = control-ref of="Lab-2"() -> (w67:refnum<vi>)
    n147 = control-ref of="Attempt-1"() -> (w81:refnum<vi>)
    n148 = control-ref of="Attempt-2"() -> (w80:refnum<vi>)
    n149 = control-ref of="Attempt-3"() -> (w79:refnum<vi>)
    n150 = control-ref of="Attempt-4"() -> (w78:refnum<vi>)
    n151 = property on="Property Node" class="Bool (strict)"(reference=w81, error in=w66, "Blinking"=w77) -> (error out=w73:errorcluster)  [unwired: 1 out]
    n152 = property on="Property Node" class="Bool (strict)"(reference=w80, error in=w66, "Blinking"=w76) -> (error out=w72:errorcluster)  [unwired: 1 out]
    n153 = property on="Property Node" class="Bool (strict)"(reference=w79, error in=w66, "Blinking"=w75) -> (error out=w71:errorcluster)  [unwired: 1 out]
    n154 = property on="Property Node" class="Bool (strict)"(reference=w78, error in=w66, "Blinking"=w74) -> (error out=w70:errorcluster)  [unwired: 1 out]
    n155 = property on="Property Node" class="Bool (strict)"(reference=w68, error in=w66, "Blinking"=w65) -> (error out=w63:errorcluster)  [unwired: 1 out]
    n156 = property on="Property Node" class="Bool (strict)"(reference=w67, error in=w66, "Blinking"=w64) -> (error out=w62:errorcluster)  [unwired: 1 out]
    n157 = Merge Errors "Merge Errors"(w73, w72, w71, w70, w63, w62) -> (w69:errorcluster)
    n158 = in-place {
      in-place-border: w69 -> [w99]
      w101 = AutocrossState."ProgramStop"  # t
      n159 = in-place-cluster #13(w92) -> ("State"=w103:T3)
      n160 = Or(x="Stop", y=w99) -> (x .or. y?=w100:bool)
      n161 = Select(t=w101, s=w100, f=w103) -> (s? t:f=w102:T3)
      n162 = in-place-cluster #13("State"=w102) -> (w91:T4)
    }
    n163 = Wait Until Next ms Multiple(millisecond multiple=w83) -> ()  [unwired: 1 out]
    n164 = Unbundle By Name(w91) -> ("CurrentRecordIndicator"=→"CurrentRecordIndicator":T1, "BestRecordIndicator"=→"BestRecordIndicator":T2)
  }
  n165 = flat-sequence {
    tunnel: w8 -> [w390]
    frame #0 {
      # "Finalized"
      n166 = call <vilib>:"Simple Error Handler.vi"("error in (no error)"=w390) -> ()  [unwired: 4 in, 5 out]
    }
  }
